vi "Scrape Screenpops.vi"(8 "error in":errorcluster, 11 "SR number list in":i32[](array[numeric])) -> (0 "error out":errorcluster, 3 "sr clusters out":T2[](array[typedef]) {"Creation Date" format="%<%x>T"; "Last Updated" format="%<%x>T"})   [LabVIEW 2018]
uses:
  <vilib>/httpClient/LabVIEWHTTPClient.lvlib
  Type Defs/SR Status.ctl
  Type Defs/SR Cluster.ctl
  Type Defs/SR Note Cluster.ctl
panel:
  out "body":string
  out "sr notes array out":T1[][](array[typedef]) {"Note Date" format="%<%x >T"}
  out "SR Note Array":T1[](array[typedef]) {"Note Date" format="%<%x >T"}
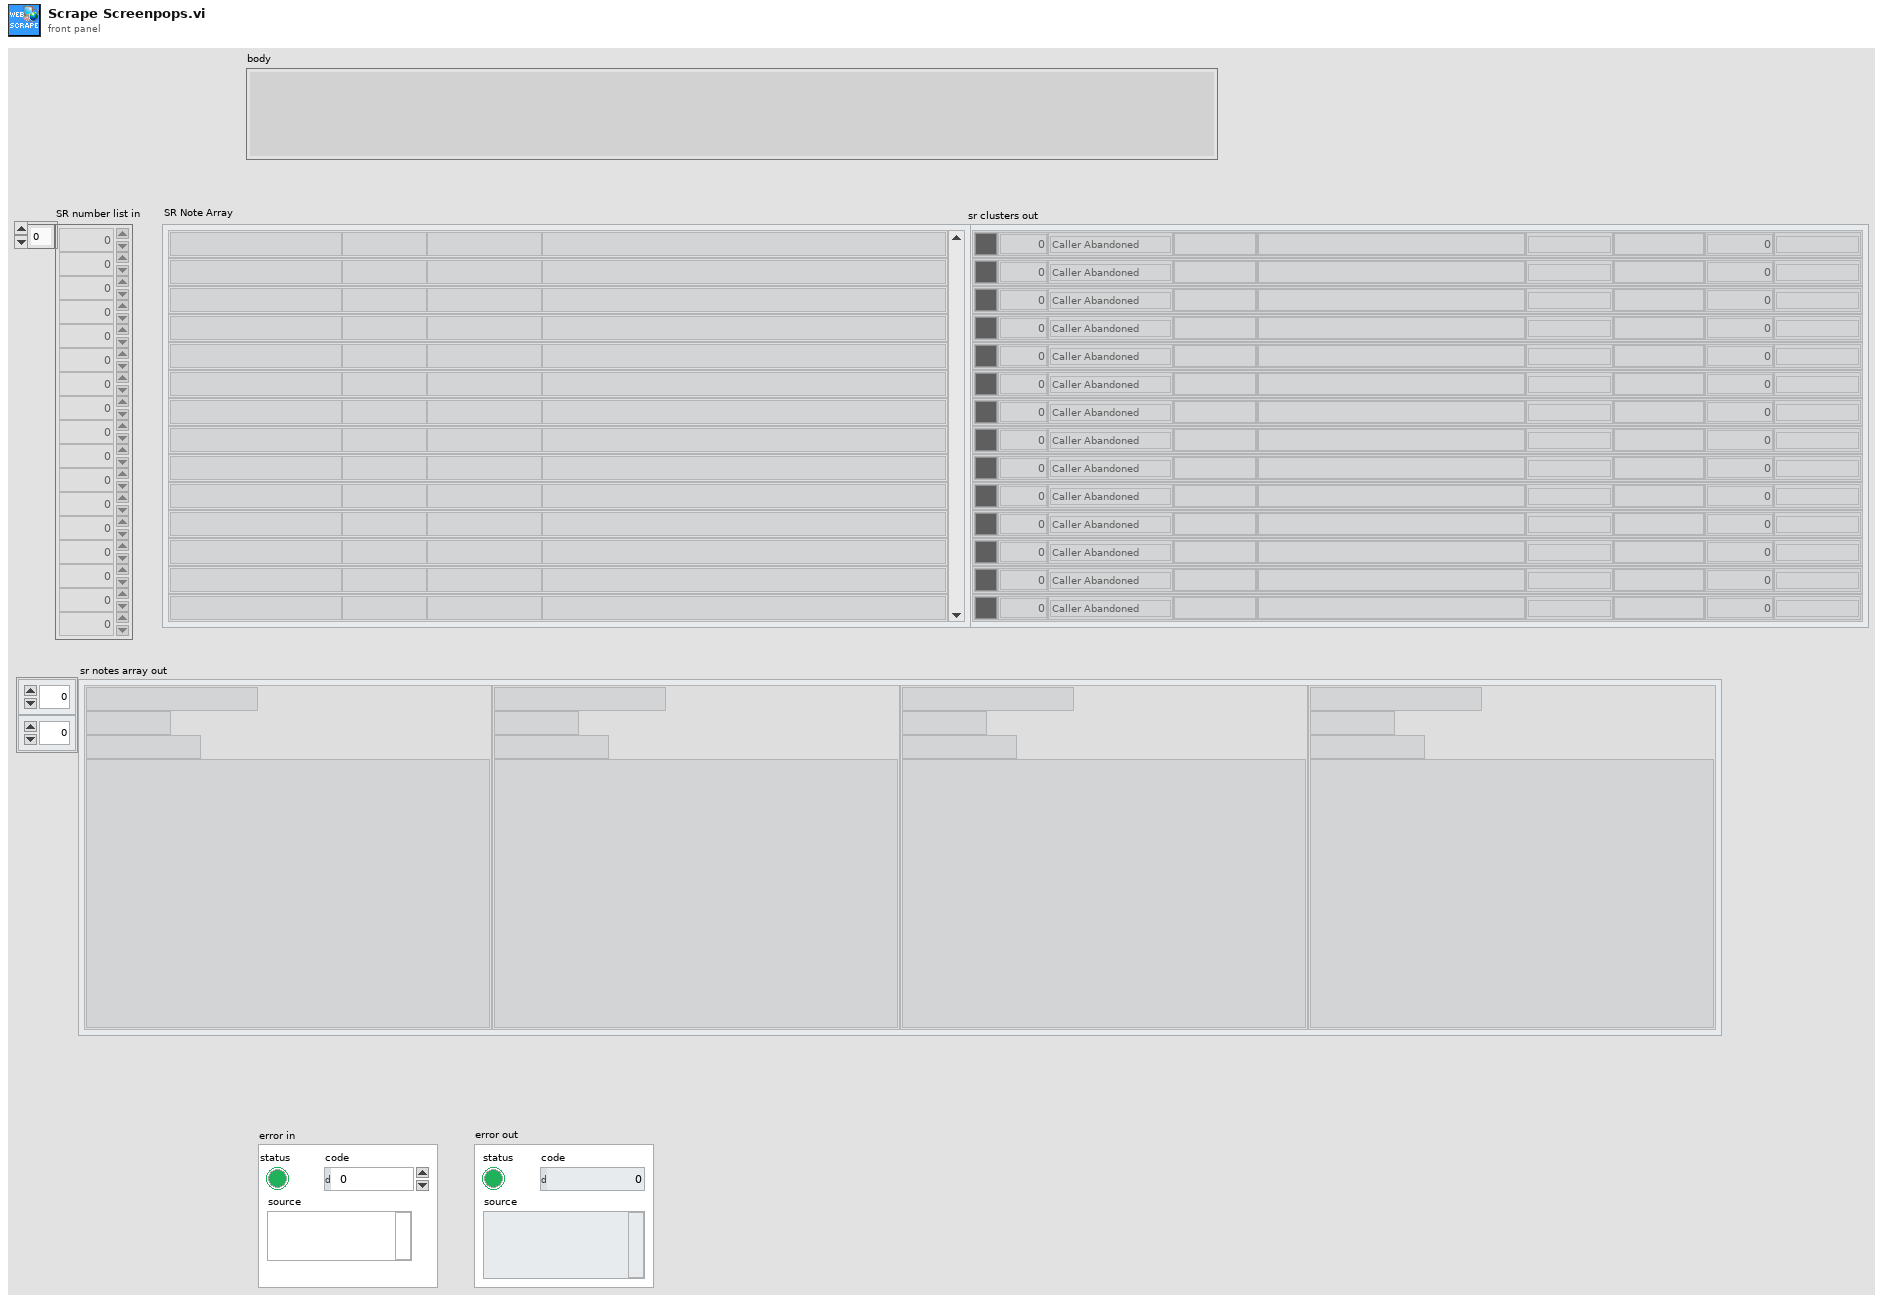
[diagram p1: front panel]
types:
  T1 = typedef "SR Note Cluster.ctl" = cluster{"Note Type":string, "Note Date":timestamp, "AE":string, "Note Text":string}
  T2 = typedef "SR Cluster.ctl" = cluster{"Color":u32, "SR Number":i32, "SR Status":T3, "SR Type":string, "Summary":string, "Last Updated":timestamp, "Service Level":string, "Days Open":dbl, "Creation Date":timestamp}
  T3 = typedef "SR Status.ctl" = enum16{"Caller Abandoned", "Created in Error", "Expired", "Forum Resolved AE", "Forum Resolved Customer", "IN WORK", "IN WORK Collab with AES", "IN WORK Collab with PSE", "IN WORK Collab with SE", "IN WORK Customer Added Note", "IN WORK Escalation", "IN WORK Wait on Customer", "Open", "Potentially Resolved", "Presumed Resolved", "RMA Approved for Return", "Resolved", "Passed Off"}
  T4 = typedef "LabVIEWHTTPClient.lvlib/ClientHandle.ctl" = refnum<k1>
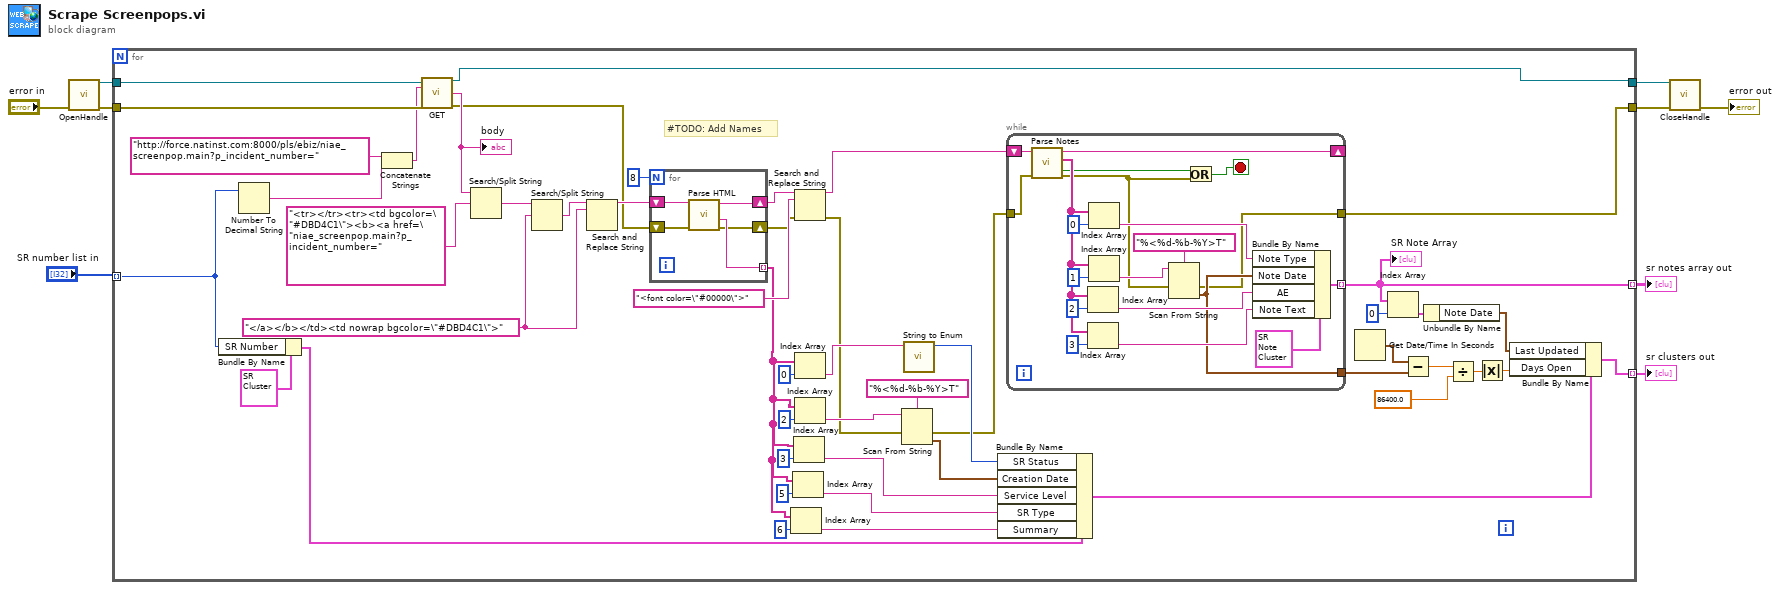
[diagram p0: block diagram]
diagram:
  n1 = call <vilib>:"OpenHandle.vi"("error in (no error)"="error in") -> ("client handle out"=w9:T4, "error out"=w8:errorcluster)  [unwired: 13 in]
  n2 = for {
    tunnel: "SR number list in" -> [w27] mode=indexing
    tunnel: [w30] -> w5 mode=indexing
    tunnel: w8 -> [w58]
    tunnel: [w24] -> w6
    tunnel: w9 -> [w59]
    tunnel: [w26] -> w7
    tunnel: [w23] -> w1 mode=indexing
    w51 = "</a></b></td><td nowrap bgcolor=\"#DBD4C1\">" ("search string/char (-)")
    # "#TODO: Add Names"
    n3 = Bundle By Name(cluster=T2 {"Color"=0, "SR Number"=0, "SR Status"=enum."Caller Abandoned", "SR Type"="", "Summary"="", "Last Updated"=timestamp(0 s since 1904-01-01), "Service Level"="", "Days Open"=0.0, "Creation Date"=timestamp(0 s since 1904-01-01)} ("SR Cluster"), "SR Number"=w27) -> (w35:T2)
    n4 = Number To Decimal String(number=w27) -> (decimal integer string=w57:string)  [unwired: 1 in]
    n5 = Concatenate Strings("http://force.natinst.com:8000/pls/ebiz/niae_screenpop.main?p_incident_number=" ("string"), w57) -> (w56:string)
    n6 = call <vilib>:"GET.vi"("client handle"=w59, "url"=w56, "error in (no error)"=w58) -> ("client handle out"=w26:T4, "body"=w55:string, "error out"=w29:errorcluster)  [unwired: 9 in, 1 out]
    "body" <- w55
    n7 = Search/Split String(string=w55, search string/char (-)="<tr></tr><tr><td bgcolor=\"#DBD4C1\"><b><a href=\"niae_screenpop.main?p_incident_number=") -> (match + rest of string=w48:string)  [unwired: 1 in, 2 out]
    n8 = Search/Split String(string=w48, search string/char (-)=w51) -> (match + rest of string=w50:string)  [unwired: 1 in, 2 out]
    n9 = Search and Replace String(input string=w50, search string=w51) -> (result string=w52:string)  [unwired: 6 in, 3 out]
    n10 = for {
      N: 8 -> [_]
      shift-right: [w63] -> w10
      shift-left: w52 -> [w64]
      tunnel: [w62] -> w39 mode=indexing
      shift-right: [w61] -> w15
      shift-left: w29 -> [w60]
      n11 = call "Parse HTML.vi"("error in"=w60, "result string in"=w64) -> ("error out"=w61:errorcluster, "data"=w62:string, "result string out"=w63:string)  [unwired: 7 in]
    }
    n12 = Index Array(array=w39, index=6) -> (element=w36:string)
    n13 = Index Array(array=w39, index=5) -> (element=w37:string)
    n14 = Index Array(array=w39, index=3) -> (element=w38:string)
    n15 = Search and Replace String(input string=w10, search string="<font color=\"#00000\">", error in=w15) -> (result string=w13:string, error out=w14:errorcluster)  [unwired: 5 in, 2 out]
    n16 = Index Array(array=w39, index=0) -> (element=w44:string)
    n17 = Index Array(array=w39, index=2) -> (element=w33:string)
    n18 = Scan From String(format string="%<%d-%b-%Y>T", input string=w33, error in=w14) -> (error out=w28:errorcluster, output 1=w32:timestamp)  [unwired: 2 in, 2 out]
    n19 = call "String to Enum.vi"("string in"=w44) -> ("enum out"=w43:T3)  [unwired: 9 in, 1 out]
    n20 = Bundle By Name(cluster=w35, "SR Status"=w43, "Creation Date"=w32, "Service Level"=w38, "SR Type"=w37, "Summary"=w36) -> (w31:T2)
    n21 = while {
      shift-right: [w83] -> _
      shift-left: w13 -> [w84]
      tunnel: w28 -> [w82]
      tunnel: [w68] -> w24
      tunnel: [w70] -> w23 mode=indexing
      tunnel: [w69] -> w18
      stop <- w67 stop-if-true
      n22 = call "Parse Notes.vi"("error in"=w82, "String"=w84) -> ("error out"=w65:errorcluster, "Done Reading?"=w66:bool, "sr note out"=w81:string[], "result string out"=w83:string)  [unwired: 6 in]
      n23 = Index Array(array=w81, index=2) -> (element=w74:string)
      n24 = Index Array(array=w81, index=3) -> (element=w75:string)
      n25 = Index Array(array=w81, index=0) -> (element=w72:string)
      n26 = Index Array(array=w81, index=1) -> (element=w71:string)
      n27 = Scan From String(format string="%<%d-%b-%Y>T", input string=w71, error in=w65) -> (error out=w68:errorcluster, output 1=w69:timestamp)  [unwired: 2 in, 2 out]
      n28 = Or(x=w66, y=w65) -> (x .or. y?=w67:bool)
      n29 = Bundle By Name(cluster=T1 {"Note Type"="", "Note Date"=timestamp(0 s since 1904-01-01), "AE"="", "Note Text"=""} ("SR Note Cluster"), "Note Type"=w72, "Note Date"=w69, "AE"=w74, "Note Text"=w75) -> (w70:T1)
    }
    "SR Note Array" <- w23
    n30 = Get Date/Time In Seconds() -> (seconds since 1Jan1904=w19:timestamp)
    n31 = Index Array(array=w23, index=0) -> (element=w21:T1)
    n32 = Subtract(x=w19, y=w18) -> (x-y=w17:dbl)
    n33 = Unbundle By Name(w21) -> ("Note Date"=w20:timestamp)
    n34 = Divide(x=w17, y=86400.0) -> (x/y=w12:dbl)
    n35 = Absolute Value(x=w12) -> (abs(x)=w11:dbl)
    n36 = Bundle By Name(cluster=w31, "Last Updated"=w20, "Days Open"=w11) -> (w30:T2)
  }
  "sr clusters out" <- w5
  "sr notes array out" <- w1
  n37 = call <vilib>:"CloseHandle.vi"("client handle"=w7, "error in (no error)"=w6) -> ("error out"=→"error out":errorcluster)  [unwired: 13 in]
